vi "SPECTRUM Set Settings_AS1.vi"(2 "error in (no error)":errorcluster, 3 "Cluster":T1 {"verticalUnit" items=["SpectrumVerticalUnit_dBm", "SpectrumVerticalUnit_Watt", "SpectrumVerticalUnit_Volt", "SpectrumVerticalUnit_Amp", "SpectrumVerticalUnit_dBmV"]; "window" items=["SpectrumWindow_Kaiser", "SpectrumWindow_Mil6dB", "SpectrumWindow_BlackmanHarris", "SpectrumWindow_Rectangle", "SpectrumWindow_FlatTop", "SpectrumWindow_Hann"]}) -> (0 "error out":errorcluster, 1 "function return":u32(ring))   [LabVIEW 2016]
doc: "RSA_API_DLL ReturnStatus SPECTRUM_SetSettings(Spectrum_Settings settings);"
uses:
  <userlib>/RSA_API/RSA_API.lvlib
  Tektronix/RSA_API/lib/x86/RSA_API.dll
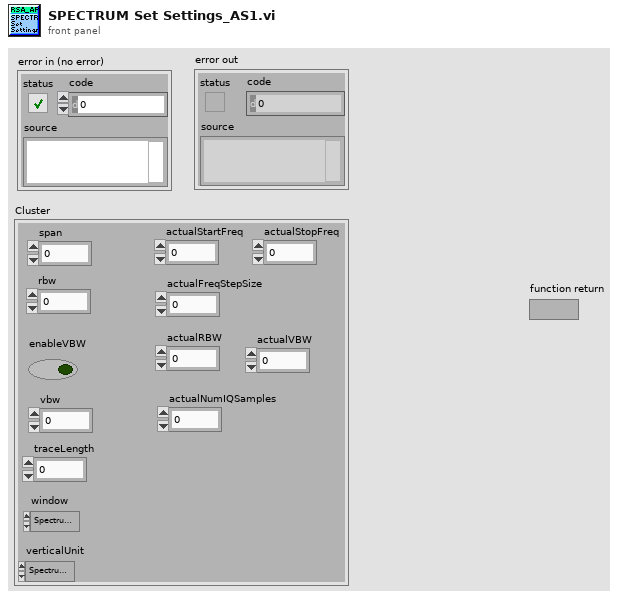
[diagram p1: front panel]
types:
  T1 = cluster{"span":dbl, "rbw":dbl, "enableVBW":bool, "vbw":dbl, "traceLength":i32, "window":u32, "verticalUnit":u32, "actualStartFreq":dbl, "actualStopFreq":dbl, "actualFreqStepSize":dbl, "actualRBW":dbl, "actualVBW":dbl, "actualNumIQSamples":i32}
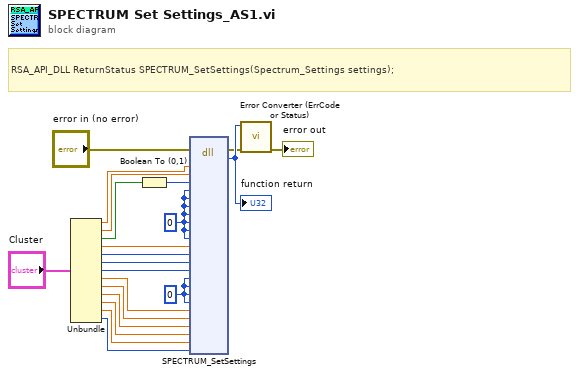
[diagram p0: block diagram]
diagram:
  w1 = i8 0 ("@dummy control@")
  w2 = i8 0 ("@dummy control@")
  # "RSA_API_DLL ReturnStatus SPECTRUM_SetSettings(Spectrum_Settings settings);"
  n1 = Unbundle("Cluster") -> ("span"=w16:dbl, "rbw"=w15:dbl, "enableVBW"=w14:bool, "vbw"=w13:dbl, "traceLength"=w12:i32, "window"=w11:u32, "verticalUnit"=w10:u32, "actualStartFreq"=w9:dbl, "actualStopFreq"=w8:dbl, "actualFreqStepSize"=w7:dbl, "actualRBW"=w6:dbl, "actualVBW"=w5:dbl, "actualNumIQSamples"=w4:i32)
  n2 = Boolean To (0,1)(Boolean=w14) -> (0, 1=w20:i16)
  n3 = dll-call lib="C:/Tektronix/RSA_API/lib/x86/RSA_API.dll" fn="SPECTRUM_SetSettings"(error in="error in (no error)", "span"=w16, "rbw"=w15, "enableVBW"=w20, "@dummy control@"=w2, "@dummy control@"=w2, "@dummy control@"=w2, "@dummy control@"=w2, "@dummy control@"=w2, "@dummy control@"=w2, "@dummy control@"=w2, "vbw"=w13, "traceLength"=w12, "window"=w11, "verticalUnit"=w10, "@dummy control@"=w1, "@dummy control@"=w1, "@dummy control@"=w1, "@dummy control@"=w1, "actualStartFreq"=w9, "actualStopFreq"=w8, "actualFreqStepSize"=w7, "actualRBW"=w6, "actualVBW"=w5, "actualNumIQSamples"=w4) -> (error out=w19:errorcluster, "return type"=w21:u32)  [unwired: 26 in, 1 out]
  "function return" <- w21
  n4 = call <userlib>:"Error Converter (ErrCode or Status).vi"("error in (no error)"=w19, "error code"=w21) -> ("error out"=→"error out":errorcluster)  [unwired: 9 in]
